vi "Speech-Status.vi"(8 "error in (no error)":errorcluster, 11 "speech_voice_refs":T1) -> (0 "error out":errorcluster, 2 "Status (T: Done)":bool, 3 "speech_voice_refs (out)":T1)   [LabVIEW 8.6]
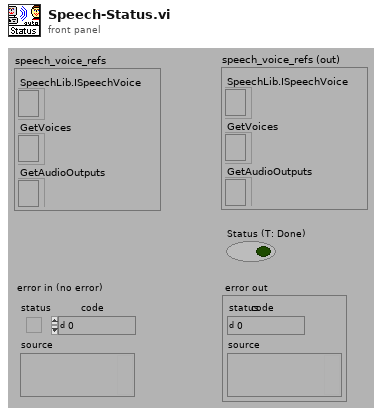
[diagram p1: front panel]
types:
  T1 = cluster{"SpeechLib.ISpeechVoice":refnum<k7>, "GetVoices":refnum<k7>, "GetAudioOutputs":refnum<k7>}
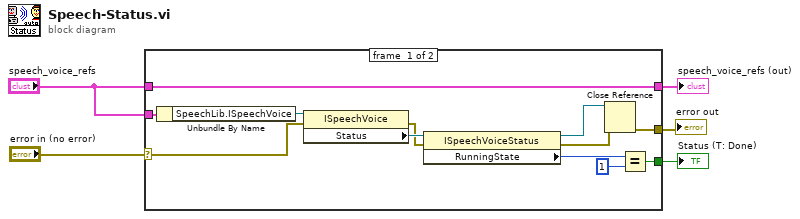
[diagram p0: block diagram]
diagram:
  n1 = case shown="No Error" "error in (no error)" {
    selector: "error in (no error)" -> [w7 w18]
    tunnel: [w17 _] -> w5
    tunnel: [w10 w18] -> w4
    tunnel: "speech_voice_refs" -> [w9 _]
    tunnel: [w6 _] -> w1
    tunnel: "speech_voice_refs" -> [w6 _]
    frame #0 {
      n2 = Unbundle By Name(w9) -> ("SpeechLib.ISpeechVoice"=w8:refnum<k7>)
      n3 = property class="ISpeechVoice"(reference=w8, error in=w7) -> (error out=w11:errorcluster, "Status"=w14:refnum<k7>)  [unwired: 1 out]
      n4 = property class="ISpeechVoiceStatus"(reference=w14, error in=w11) -> (reference out=w13:refnum<k7>, error out=w12:errorcluster, "RunningState"=w15:i32)
      n5 = Close Reference(reference=w13, error in (no error)=w12) -> (error out=w10:errorcluster)
      n6 = Equal?(x=w15, y=1) -> (x = y?=w17:bool)
    }
    frame #1 {
    }
  }
  "Status (T: Done)" <- w5
  "error out" <- w4
  "speech_voice_refs (out)" <- w1
